vi "Wait for LVx Response via Notifier.vi"(0 "response notifier":T1, 9 "timeout in ms (10000)":i32=10000, 11 "error in":errorcluster) -> (4 "data":refnum<class "LVx.lvclass">, 10 "timed out?":bool, 15 "error out":errorcluster)   [LabVIEW 2011, in "LVx.lvlib" / "LVx.lvclass"]
uses:
  LVx.lvclass
  TypeDef/Typedef - LVx Response Notifier.ctl
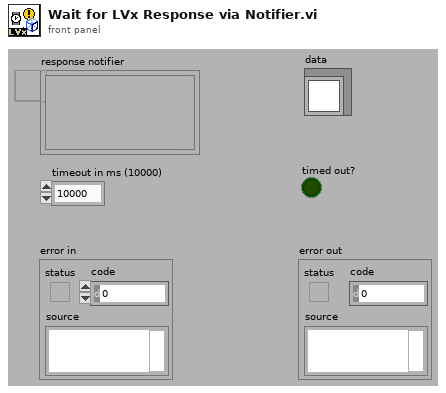
[diagram p1: front panel]
types:
  T1 = typedef "LVx.lvlib/LVx.lvclass/Typedef - LVx Response Notifier.ctl" = refnum<notifier>
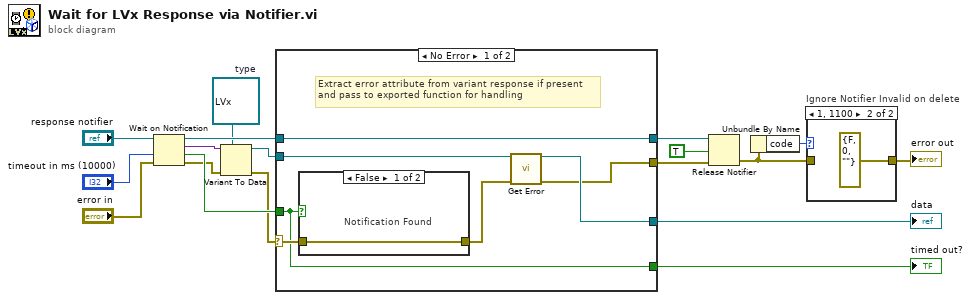
[diagram p0: block diagram]
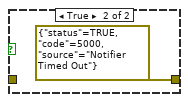
[diagram p3: hidden frame]
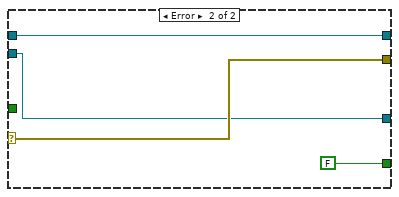
[diagram p4: hidden frame]
diagram:
  w1 = refnum<class "LVx.lvclass"> refnum  # type
  n1 = Wait on Notification(notifier="response notifier", timeout in ms (-1)="timeout in ms (10000)", error in (no error)="error in") -> (notifier out=w15:T1, notification=w8:variant, timed out?=w12:bool, error out=w2:errorcluster)  [unwired: 1 out]
  n2 = Variant To Data(error in=w2, type=w1, Variant=w8) -> (data=w7:refnum<class "LVx.lvclass">, error out=w3:errorcluster)
  n3 = case shown="No Error" w3 {
    selector: w3 -> [w24 w30]
    tunnel: w7 -> [w22 w29]
    tunnel: [w20 w29] -> w10
    tunnel: [w19 w30] -> w16
    tunnel: w15 -> [w25 w31]
    tunnel: [w25 w31] -> w17
    tunnel: w12 -> [w23 _]
    tunnel: [w23 FALSE ("timed out?")] -> w11
    frame No Error {
      # "Extract error attribute from variant response if present\nand pass to exported function for handling"
      n4 = case shown="False" w23 {
        tunnel: [w26 errorcluster {"status"=TRUE, "code"=5000, "source"="Notifier Timed Out"} ("error out")] -> w21
        tunnel: w24 -> [w26 _]
        frame False {
          # "Notification Found"
        }
        frame True {
        }
      }
      n5 = call "Get Error.vi"("LVx.lvlib:LVx.lvclass"=w22, "error in (no error)"=w21) -> ("LVx.lvlib:LVx.lvclass 2"=w20:refnum<class "LVx.lvclass">, "error out"=w19:errorcluster)  [unwired: 12 out]
    }
    frame Error {
    }
  }
  "data" <- w10
  "timed out?" <- w11
  n6 = Release Notifier(notifier=w17, force destroy? (F)=TRUE, error in (no error)=w16) -> (error out=w4:errorcluster)  [unwired: 2 out]
  n7 = Unbundle By Name(w4) -> ("code"=w6:i32)
  n8 = case "Ignore Notifier Invalid on delete" shown="1, 1100" w6 {
    tunnel: w4 -> [w32 _]
    tunnel: [w32 errorcluster {"status"=FALSE, "code"=0, "source"=""} ("error out")] -> w5
    frame Default {
    }
    frame 1, 1100 {
    }
  }
  "error out" <- w5
